vi "Add Variables to RD header.vi"() -> (4 "Path":path)   [LabVIEW 2020]
panel:
  out "Values":string[](array[string])
  out "Name":string[](array[string])
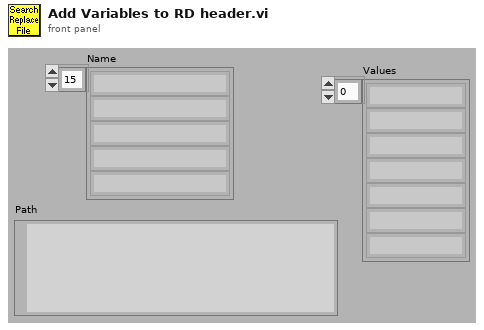
[diagram p1: front panel]
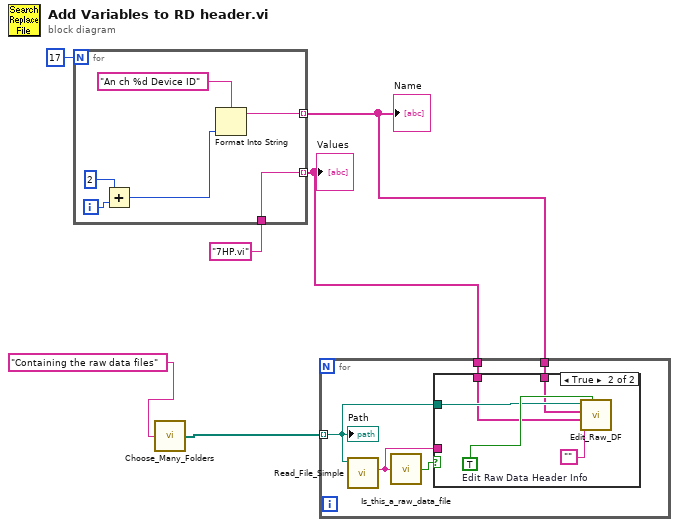
[diagram p0: block diagram]
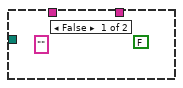
[diagram p2: hidden frame]
diagram:
  n1 = for {
    N: 17 -> [_]
    tunnel: [w8] -> w2 mode=indexing
    tunnel: [w7] -> w1 mode=indexing
    tunnel: "7HP.vi" -> [w7]
    i -> [w12]
    n2 = Add(x=2, y=w12) -> (x+y=w9:i32)
    n3 = Format Into String(format string="An ch %d Device ID", w9) -> (resulting string=w8:string)  [unwired: 2 in, 1 out]
  }
  "Name" <- w2
  "Values" <- w1
  n4 = call "Choose_Many_Folders.vi"("Purpose of choosing folder"="Containing the raw data files") -> ("Files"=w3:path[])
  n5 = for {
    tunnel: w3 -> [w15] mode=indexing
    tunnel: w2 -> [w14]
    tunnel: w1 -> [w13]
    n6 = call "Read_File_Simple.vi"("Filename"=w15) -> ("string"=w17:string)  [unwired: 4 in, 5 out]
    n7 = call "Is_this_a_raw_data_file.vi"("character string"=w17) -> ("Raw Dat File?"=w16:bool)  [unwired: 2 out]
    n8 = case shown="True" w16 {
      tunnel: w17 -> [_ _]
      tunnel: w15 -> [_ w21]
      tunnel: w14 -> [_ w20]
      tunnel: w13 -> [_ w19]
      frame False {
        (unwired) "" ("string")
        (unwired) FALSE
      }
      frame True {
        w22 = TRUE  # Edit Raw Data Header Info
        n9 = call "Edit_Raw_DF.vi"("Edit Raw Data Header Info"=w22, "New Analysis Info Cluster Setup"="", "New Values In"=w19, "New Chs In"=w20, "Data filename"=w21) -> ()  [unwired: 1 in, 4 out]
      }
    }
    "Path" <- w15
  }
